vi "AP2_scope_viewer.vi"() -> ()   [LabVIEW 2023]
uses:
  <instrlib>/niScope/Controls/niScope vertical coupling.ctl
  <instrlib>/niScope/Controls/niScope trigger slope.ctl
  <instrlib>/niScope/Controls/niScope trigger source.ctl
panel:
  in  "Tab Control 2":enum32{"General", "Monitoring", "Advanced"}(tab)
  in  "stop":bool
  in  "Save C1 Trace":bool
  in  "Save C2 Trace":bool
  in  "C1 enabled":bool=TRUE caption="Enabled?"
  in  "C2 enabled":bool=TRUE caption="Enabled?"
  in  "Reset Summed Averages":bool
  in  "RT Avg Trace #":i32=10 min=1
  in  "Summed Trace #":i32=1000 min=1
  in  "Trigger delay / us":dbl caption="trigger delay" format="%.5f"
  in  "Probe Duration / us":dbl=100.0
  in  "Samples":i64(ring)=500000 items=["500 S"=500, "1 kS"=1000, "5 kS"=5000, "10 kS"=10000, "100 kS"=100000, "500 kS"=500000, "1 MS"=1000000, "2.5 MS"=2500000, "5MS"=5000000, "10 MS"=10000000, "20 MS"=20000000]
  in  "C1 Offset / V":dbl caption="vertical offset" format="%.4f"
  in  "C1 Coupling / V":T1=1 caption="vertical coupling" items=["AC", "DC", "Ground"]
  in  "C1 Range / V":dbl=0.1 caption="vertical range" min=0.1 max=5.0 step=0.1 format="%.2f"
  in  "C1 Attenuation":dbl=2.0 caption="probe attenuation" format="%.1f"
  in  "C1 Impedance":u32(ring)=2 caption="input impedance" items=["1 mega ohm"=0, "50 ohms"=2]
  in  "C2 Offset / V":dbl caption="vertical offset" format="%.4f"
  in  "C2 Range / V":dbl=1.0 caption="vertical range" min=0.1 max=5.0 step=0.1 format="%.2f"
  in  "C2 Attenuation":dbl=1.0 caption="probe attenuation" format="%.1f"
  in  "C2 Coupling / V":T1=1 caption="vertical coupling" items=["AC", "DC", "Ground"]
  in  "C2 Impedance":u32(ring)=2 caption="input impedance" items=["1 mega ohm"=0, "50 ohms"=2]
  in  "Trigger slope":T2 items=["Positive", "Negative"]
  in  "Trigger Source":string(combo)="VAL_PFI_0"
  in  "Load Scope Config":bool
  in  "Save Scope Config":bool
  out "Aqusition Time / ms":u32=100
  out "Aquisition Frequency / Hz":dbl=10.0
  out "Summed Avg  Exectuion Time / ms":u32=14
  out "Raw Data Processing  Exectuion Time / ms":u32=103
  out "RT Average Exectuion Time / ms":u32=18
  in  "Scope Channel":refnum<k15>="PXI1Slot2" caption="resource name"
  in  "Default Data Directory":path=path "" caption="start path"
  in  "C1 maximum input frequency / Hz":dbl=100.0 caption="max input frequency" format="%.2f"
  in  "Enforce realtime":bool=TRUE caption="enforce realtime"
  in  "C2 maximum input frequency / Hz":dbl caption="max input frequency" format="%.2f"
  in  "Load old conditions?":bool
  in  "Intercept":dbl
  in  "Gradient":dbl
  in  "Mass Conversion":bool
  in  "Tab Control 6":enum32{"Time Traces", "Mass Traces"}(tab)
  in  "Tab Control":T3(tab)=enum."Real Time Average Traces"
  in  "Tab Control 3":enum32{"Channel 1", "Channel 2"}(tab)
  out "Channel 2 Raw":waveform(dbl)(graph)
  out "Channel 1 Raw":waveform(dbl)(graph)
  in  "Tab Control 4":enum32{"Channel 1", "Channel 2"}(tab)
  out "Channel 1 RT Avg":waveform(dbl)(graph)
  out "Channel 2 RT Avg":waveform(dbl)(graph)
  in  "Tab Control 5":enum32{"Channel 1", "Channel 2"}(tab)
  out "Channel 1 Summed Avg":waveform(dbl)(graph)={"t0"=timestamp(3803903996.848833 s since 1904-01-01), "dt"=4e-10, "Y"=array[250000 elements]}
  out "Trace # (C1)":i32=1000
  out "Channel 2  Summed Avg":waveform(dbl)(graph)={"t0"=timestamp(3803903996.848833 s since 1904-01-01), "dt"=4e-10, "Y"=array[250000 elements]}
  out "Trace # (C2)":i32=1000
  in  "Tab Control 10":T3(tab)
  in  "Tab Control 7":enum32{"Channel 1", "Channel 2"}(tab)
  out "C1 Raw (mass)":cluster{dbl[], "Y":dbl[]}(graph)
  out "C2 Raw (mass)":cluster{dbl[], "Y":dbl[]}(graph)
  in  "Tab Control 8":enum32{"Channel 1", "Channel 2"}(tab)
  out "C1 RT avg (mass)":cluster{dbl[], "Y":dbl[]}(graph)
  out "C2 RT avg (mass)":cluster{dbl[], "Y":dbl[]}(graph)
  in  "Tab Control 9":enum32{"Channel 1", "Channel 2"}(tab)
  out "C1 Summed avg (mass)":cluster{dbl[], "Y":dbl[]}(graph)
  out "C2 Summed avg (mass)":cluster{dbl[], "Y":dbl[]}(graph)
  # "Triggering Controls"
  # "Vertical Controls"
  # "Horizontal Controls"
  # "Averaging Controls"
  # "Mass Conversion Controls"
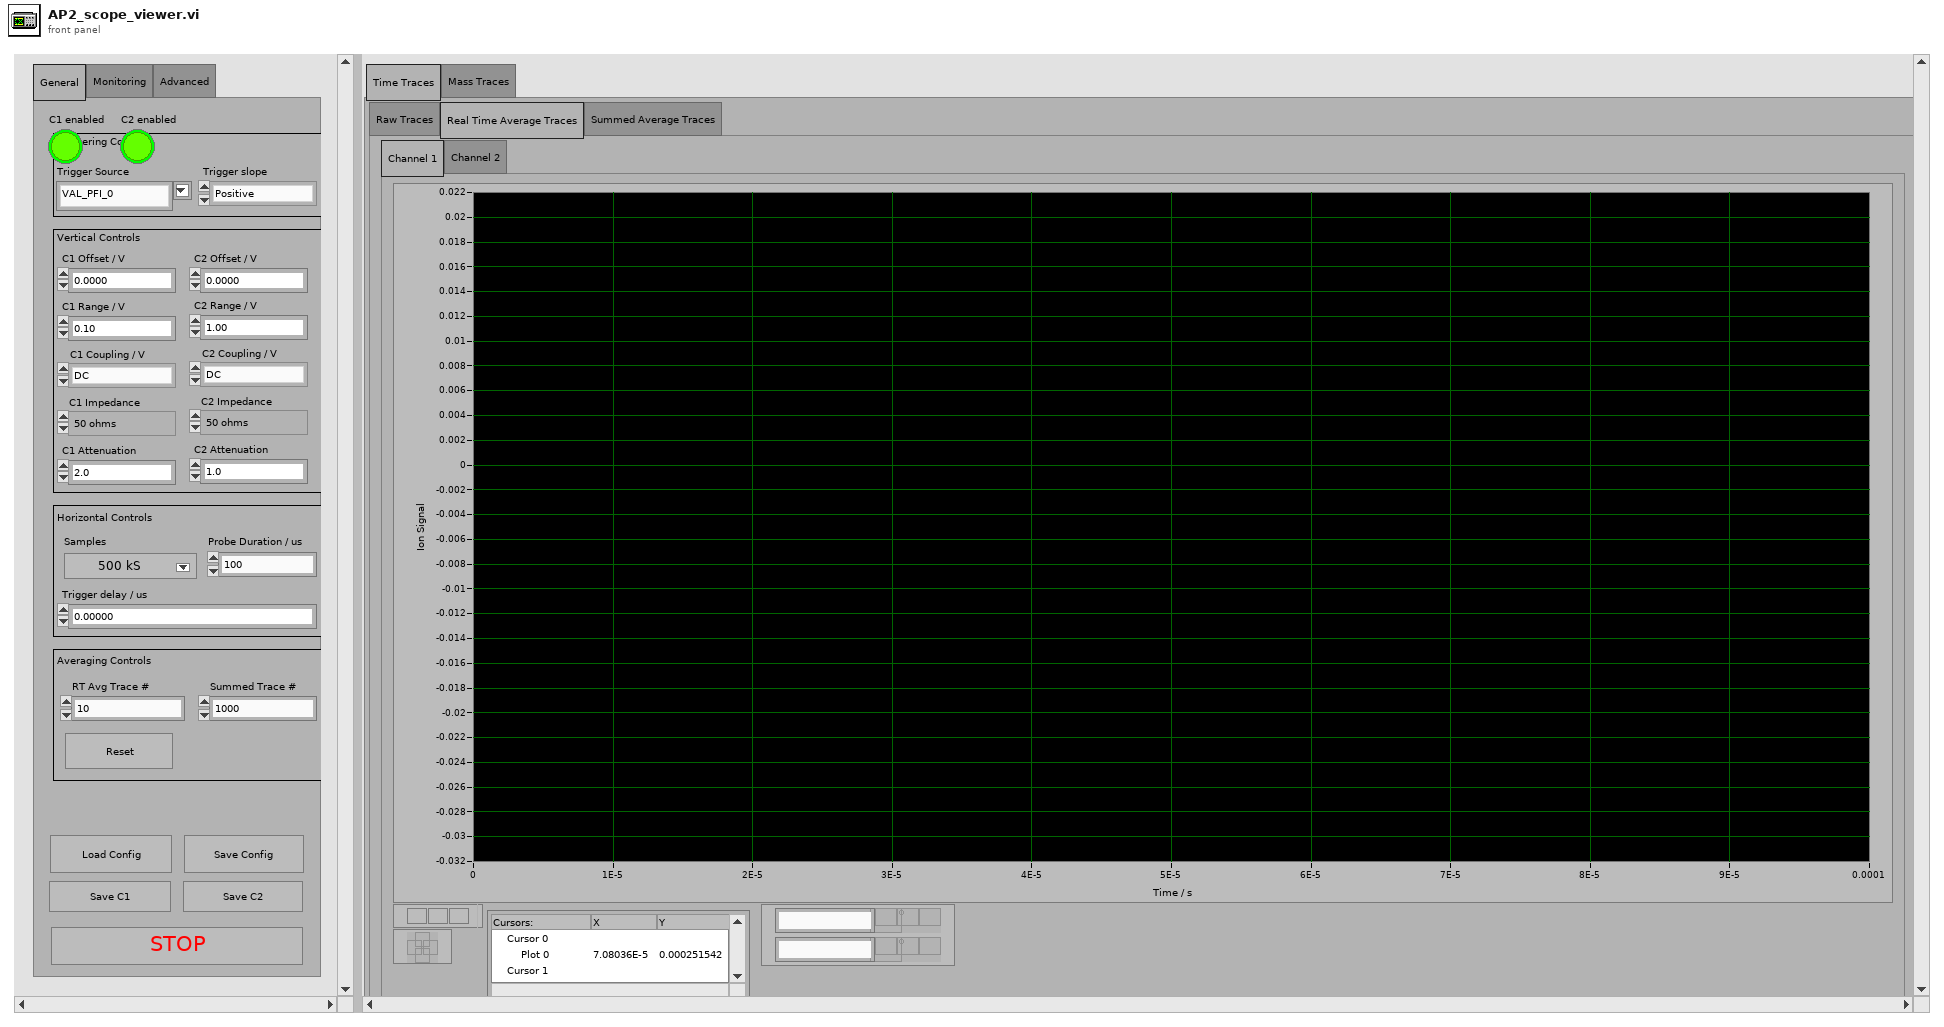
[diagram p1: front panel]
types:
  T1 = typedef "niScope vertical coupling.ctl" = i32
  T2 = typedef "niScope trigger slope.ctl" = i32
  T3 = enum32{"Raw Traces", "Real Time Average Traces", "Summed Average Traces"}
  T4 = cluster{"Trigger Source":refnum<vi>, "Trigger delay / us":refnum<vi>, "Trigger slope":refnum<vi>, "Probe Duration / us":refnum<vi>, "Samples":refnum<vi>, "Enforce realtime":refnum<vi>, "C2 Impedance":refnum<vi>, "C2 maximum input frequency / Hz":refnum<vi>, "C2 enabled":refnum<vi>, "C2 Coupling / V":refnum<vi>, "C2 Attenuation":refnum<vi>, "C2 Range / V":refnum<vi>, "C2 Offset / V":refnum<vi>, "C1 Impedance":refnum<vi>, "C1 maximum input frequency / Hz":refnum<vi>, "C1 enabled":refnum<vi>, "C1 Coupling / V":refnum<vi>, "C1 Attenuation":refnum<vi>, "C1 Range / V":refnum<vi>, "C1 Offset / V":refnum<vi>, "Scope Channel":refnum<vi>}
  T5 = cluster{"C1 Summed Waveform 2":waveform(dbl), "C1 Summed Waveform 2":waveform(dbl)}
  T6 = cluster{"Gradient":dbl, "Intercept":dbl, "RT Avg Trace #":i32, "Summed Avg Trace #":i32, "Mass Conversion":bool}
  T7 = typedef "niScope trigger source.ctl" = string
  T8 = cluster{"Scope Channel":refnum<k15>, "C1 vertical offset / V":dbl, "C1 vertical range / V":dbl, "C1 probe attenuation":dbl, "C1 vertical coupling / V":T1, "C1 enabled":bool, "C1 maximum input frequency / Hz":dbl, "C1 input impedance / ohms":u32, "C2 vertical offset / V":dbl, "C2 vertical range / V":dbl, "C2 probe attenuation":dbl, "C2 vertical coupling / V":T1, "C2 enabled":bool, "C2 maximum input frequency / Hz":dbl, "C2 input impedance / ohms":u32, "Enforce realtime":bool, "Samples":i64, "tmax / us ":dbl, "Trigger source":T7, "Trigger slope":T2, "Trigger delay / us":dbl}
  T9 = cluster{"queue out":refnum<queue>, "error out":errorcluster, "queue out":refnum<queue>, "error out":errorcluster, "queue out":refnum<queue>, "error out":errorcluster, "queue out":refnum<queue>, "error out":errorcluster}
  T10 = cluster{"queue out":refnum<queue>, "error out":errorcluster, "queue out":refnum<queue>, "error out":errorcluster}
  T11 = cluster{"output cluster":cluster{"wfm info":cluster{"actualSamples":i32, "absoluteInitialX":dbl, "relativeInitialX":dbl, "xIncrement":dbl, "offset":dbl, "gain":dbl, "reserved1":dbl, "reserved2":dbl}, "Offset WFm":waveform(dbl), bool}, "output cluster":cluster{"wfm info":cluster{"actualSamples":i32, "absoluteInitialX":dbl, "relativeInitialX":dbl, "xIncrement":dbl, "offset":dbl, "gain":dbl, "reserved1":dbl, "reserved2":dbl}, "Offset WFm":waveform(dbl), bool}}
  T12 = cluster{"Cycle Count In":i32, "Cycle Count In":i32}
  T13 = cluster{"output cluster":cluster{"wfm info":cluster{"actualSamples":i32, "absoluteInitialX":dbl, "relativeInitialX":dbl, "xIncrement":dbl, "offset":dbl, "gain":dbl, "reserved1":dbl, "reserved2":dbl}, "C1 Summed Waveform 2":waveform(dbl), bool}, "output cluster":cluster{"wfm info":cluster{"actualSamples":i32, "absoluteInitialX":dbl, "relativeInitialX":dbl, "xIncrement":dbl, "offset":dbl, "gain":dbl, "reserved1":dbl, "reserved2":dbl}, "C1 Summed Waveform 2":waveform(dbl), bool}, "C1 Mass Data":cluster{dbl, cluster{dbl, dbl}, cluster{dbl[], "Y":dbl[]}}, "C2 Mass Data":cluster{dbl, cluster{dbl, dbl}, cluster{dbl[], "Y":dbl[]}}}
  T14 = cluster{"offset":dbl, "C1 Summed Waveform 2":waveform(dbl)}
  T15 = cluster{"elements":cluster{"wfm info":cluster{"actualSamples":i32, "absoluteInitialX":dbl, "relativeInitialX":dbl, "xIncrement":dbl, "offset":dbl, "gain":dbl, "reserved1":dbl, "reserved2":dbl}, "Offset WFm":waveform(dbl), bool}[], "elements":cluster{"wfm info":cluster{"actualSamples":i32, "absoluteInitialX":dbl, "relativeInitialX":dbl, "xIncrement":dbl, "offset":dbl, "gain":dbl, "reserved1":dbl, "reserved2":dbl}, "Offset WFm":waveform(dbl), bool}[]}
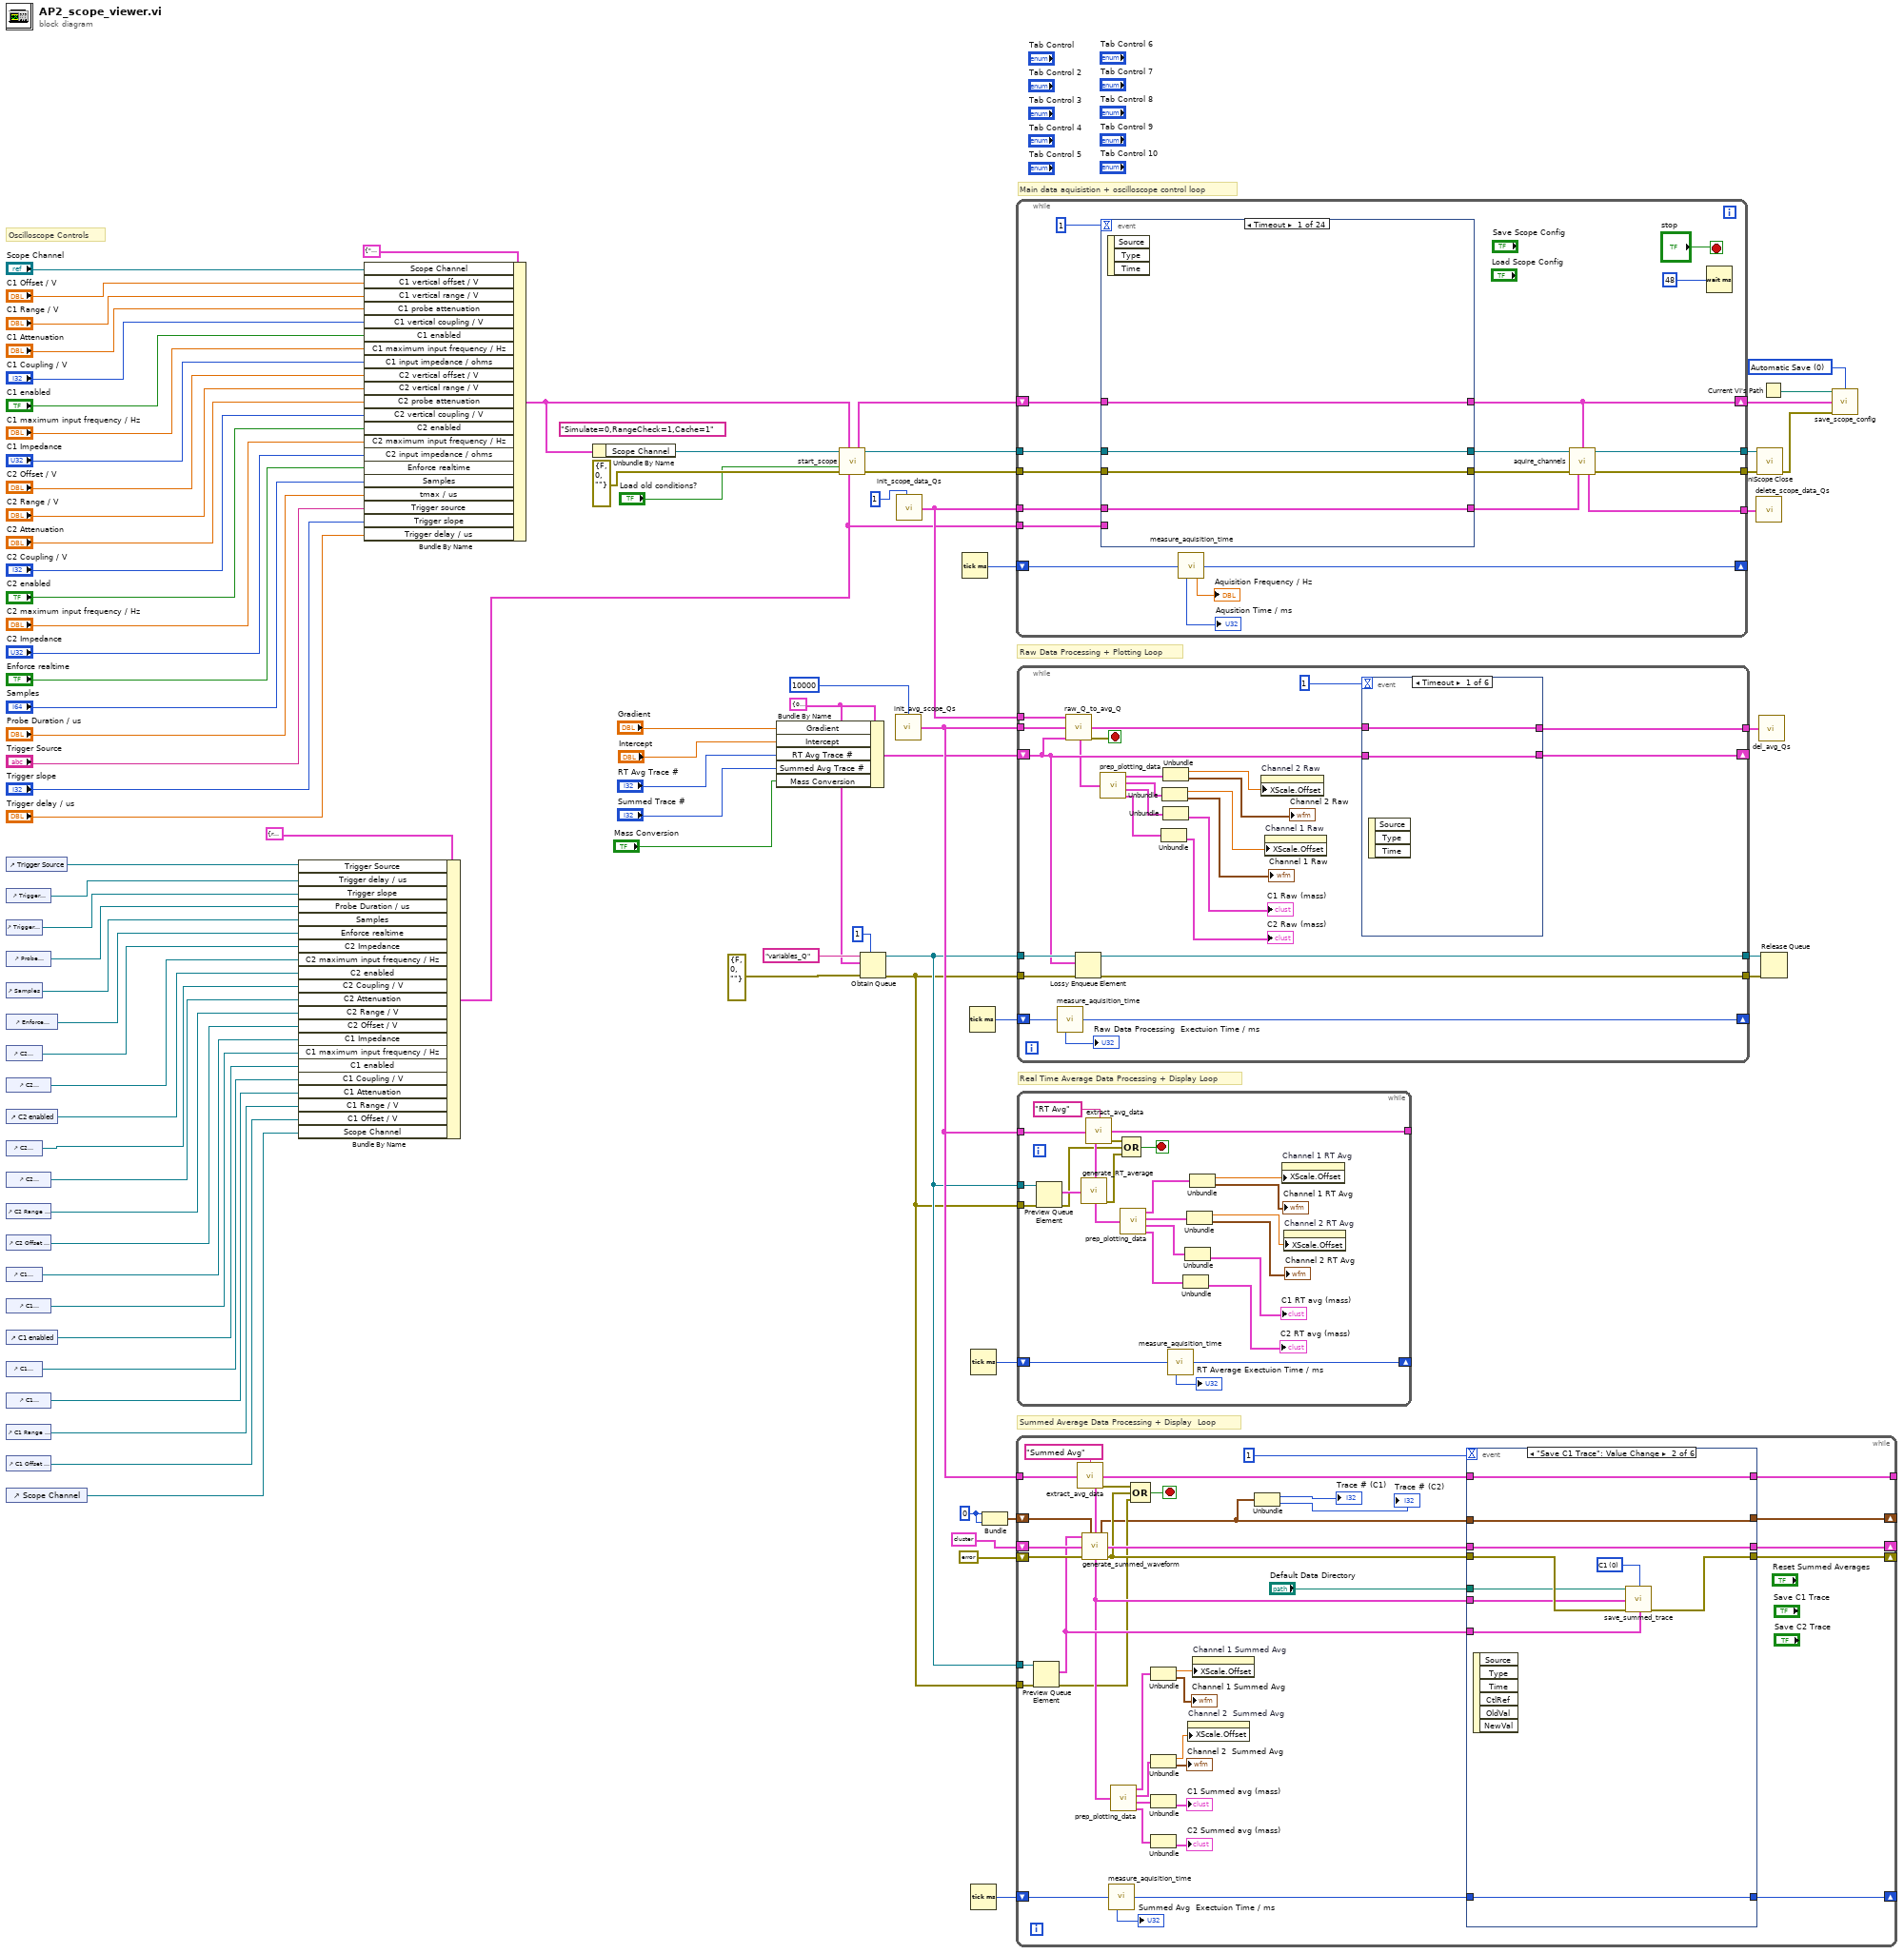
[diagram p0: block diagram]
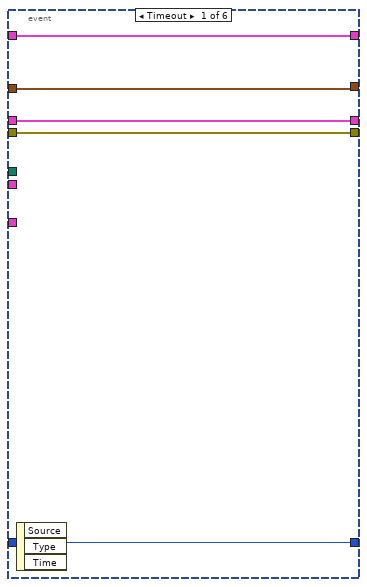
[diagram p2: hidden frame]
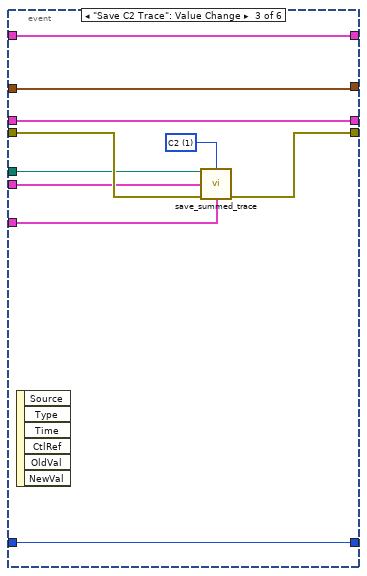
[diagram p3: hidden frame]
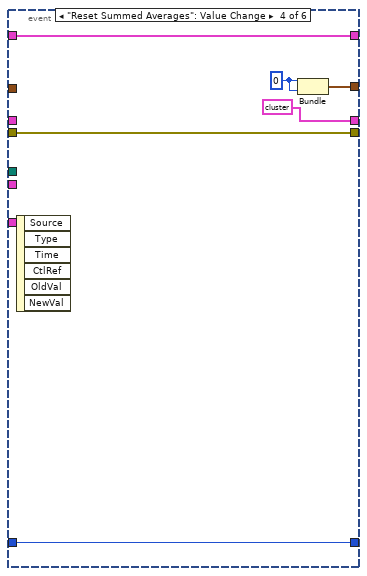
[diagram p4: hidden frame]
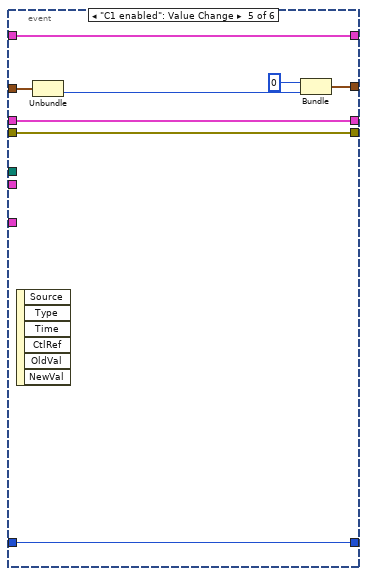
[diagram p5: hidden frame]
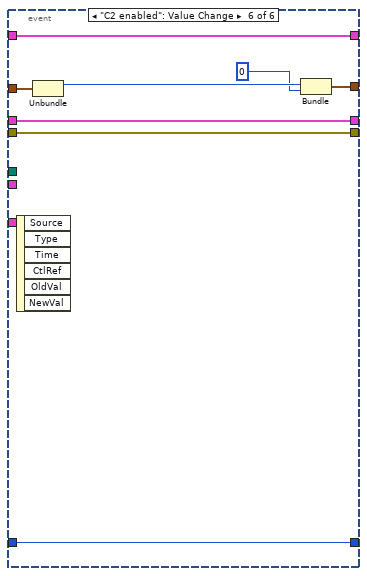
[diagram p6: hidden frame]
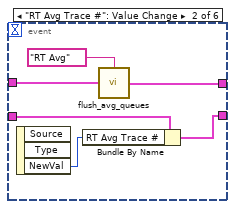
[diagram p7: hidden frame]
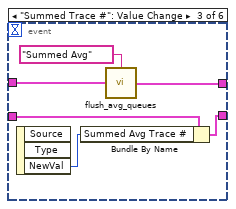
[diagram p8: hidden frame]
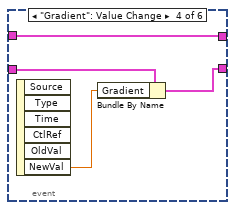
[diagram p9: hidden frame]
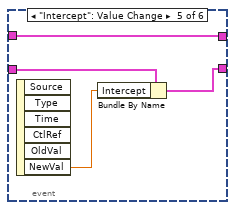
[diagram p10: hidden frame]
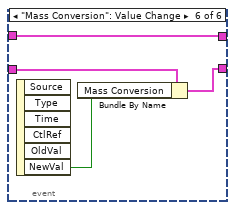
[diagram p11: hidden frame]
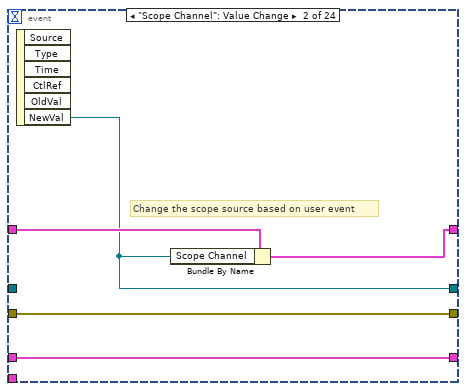
[diagram p12: hidden frame]
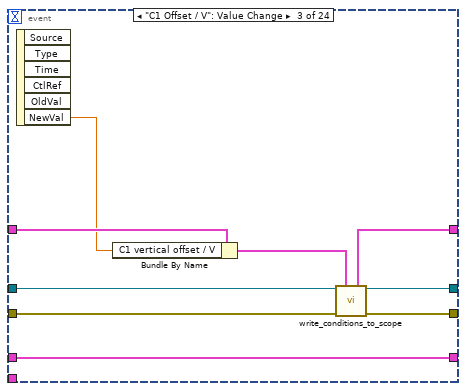
[diagram p13: hidden frame]
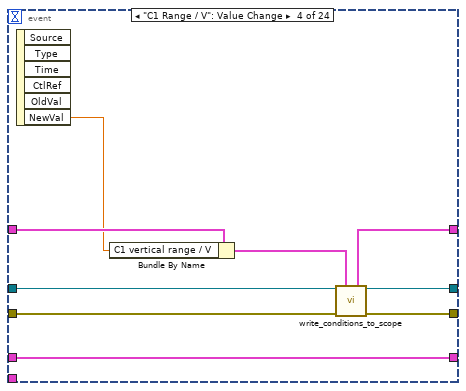
[diagram p14: hidden frame]
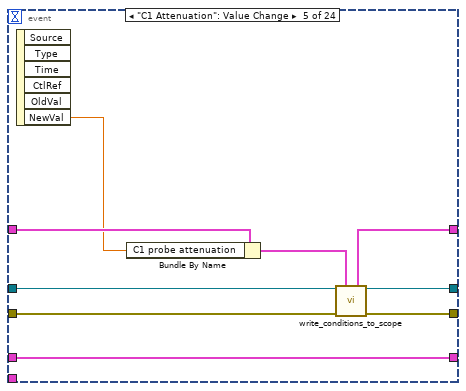
[diagram p15: hidden frame]
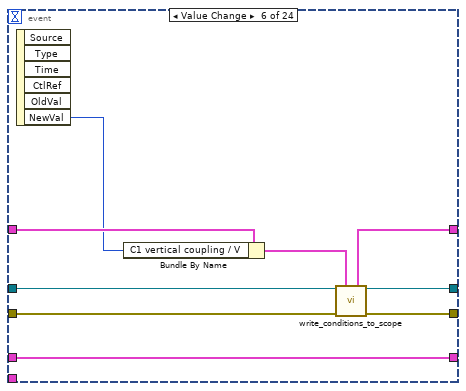
[diagram p16: hidden frame]
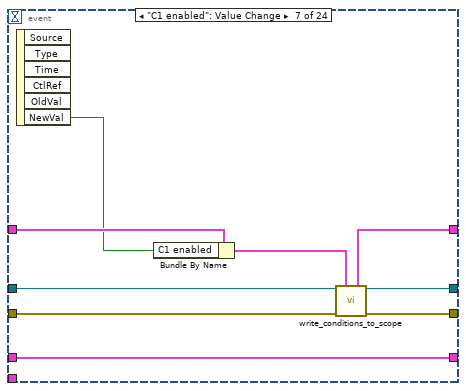
[diagram p17: hidden frame]
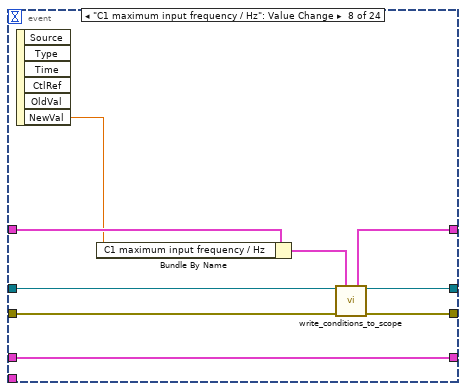
[diagram p18: hidden frame]
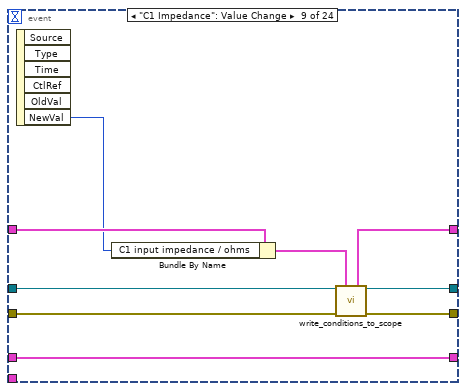
[diagram p19: hidden frame]
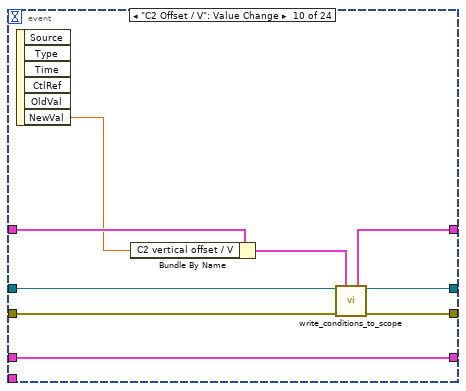
[diagram p20: hidden frame]
diagram:
  w31 = u16 0 items=["Automatic Save", "Custom File"] ("Save File Type")
  w41 = 0
  w49 = T6 {"Gradient"=0.0, "Intercept"=0.0, "RT Avg Trace #"=0, "Summed Avg Trace #"=0, "Mass Conversion"=FALSE}
  (unwired) "Simulate=0,RangeCheck=1,Cache=1" ("option string")
  # "Summed Average Data Processing + Display  Loop"
  # "Real Time Average Data Processing + Display Loop"
  # "Oscilloscope Controls"
  # "Raw Data Processing + Plotting Loop"
  # "Main data aquisistion + oscilloscope control loop"
  n1 = control-ref of="Trigger Source"() -> (w23:refnum<vi>)
  n2 = control-ref of="Trigger delay / us"() -> (w21:refnum<vi>)
  n3 = control-ref of="Trigger slope"() -> (w20:refnum<vi>)
  n4 = control-ref of="Probe Duration / us"() -> (w19:refnum<vi>)
  n5 = control-ref of="Samples"() -> (w18:refnum<vi>)
  n6 = control-ref of="Enforce realtime"() -> (w17:refnum<vi>)
  n7 = control-ref of="C2 Impedance"() -> (w16:refnum<vi>)
  n8 = control-ref of="C2 maximum input frequency / Hz"() -> (w15:refnum<vi>)
  n9 = control-ref of="C2 enabled"() -> (w14:refnum<vi>)
  n10 = control-ref of="C2 Coupling / V"() -> (w13:refnum<vi>)
  n11 = control-ref of="C2 Attenuation"() -> (w12:refnum<vi>)
  n12 = control-ref of="C2 Range / V"() -> (w11:refnum<vi>)
  n13 = control-ref of="C2 Offset / V"() -> (w10:refnum<vi>)
  n14 = control-ref of="C1 Impedance"() -> (w9:refnum<vi>)
  n15 = control-ref of="C1 maximum input frequency / Hz"() -> (w8:refnum<vi>)
  n16 = control-ref of="C1 enabled"() -> (w7:refnum<vi>)
  n17 = control-ref of="C1 Coupling / V"() -> (w6:refnum<vi>)
  n18 = control-ref of="C1 Attenuation"() -> (w5:refnum<vi>)
  n19 = control-ref of="C1 Range / V"() -> (w4:refnum<vi>)
  n20 = control-ref of="C1 Offset / V"() -> (w3:refnum<vi>)
  n21 = control-ref of="Scope Channel"() -> (w2:refnum<vi>)
  n22 = Bundle By Name(cluster=T4 {"Trigger Source"=refnum, "Trigger delay / us"=refnum, "Trigger slope"=refnum, "Probe Duration / us"=refnum, "Samples"=refnum, "Enforce realtime"=refnum, "C2 Impedance"=refnum, "C2 maximum input frequency / Hz"=refnum, "C2 enabled"=refnum, "C2 Coupling / V"=refnum, "C2 Attenuation"=refnum, "C2 Range / V"=refnum, "C2 Offset / V"=refnum, "C1 Impedance"=refnum, "C1 maximum input frequency / Hz"=refnum, "C1 enabled"=refnum, "C1 Coupling / V"=refnum, "C1 Attenuation"=refnum, "C1 Range / V"=refnum, "C1 Offset / V"=refnum, "Scope Channel"=refnum}, "Trigger Source"=w23, "Trigger delay / us"=w21, "Trigger slope"=w20, "Probe Duration / us"=w19, "Samples"=w18, "Enforce realtime"=w17, "C2 Impedance"=w16, "C2 maximum input frequency / Hz"=w15, "C2 enabled"=w14, "C2 Coupling / V"=w13, "C2 Attenuation"=w12, "C2 Range / V"=w11, "C2 Offset / V"=w10, "C1 Impedance"=w9, "C1 maximum input frequency / Hz"=w8, "C1 enabled"=w7, "C1 Coupling / V"=w6, "C1 Attenuation"=w5, "C1 Range / V"=w4, "C1 Offset / V"=w3, "Scope Channel"=w2) -> (w1:T4)
  n23 = Bundle By Name(cluster=T8 {"Scope Channel"="", "C1 vertical offset / V"=0.0, "C1 vertical range / V"=5.0, "C1 probe attenuation"=1.0, "C1 vertical coupling / V"=1, "C1 enabled"=TRUE, "C1 maximum input frequency / Hz"=0.0, "C1 input impedance / ohms"=0, "C2 vertical offset / V"=0.0, "C2 vertical range / V"=5.0, "C2 probe attenuation"=1.0, "C2 vertical coupling / V"=1, "C2 enabled"=TRUE, "C2 maximum input frequency / Hz"=0.0, "C2 input impedance / ohms"=0, "Enforce realtime"=TRUE, "Samples"=0, "tmax / us "=0.0, "Trigger source"="0", "Trigger slope"=0, "Trigger delay / us"=0.0}, "Scope Channel"="Scope Channel", "C1 vertical offset / V"="C1 Offset / V", "C1 vertical range / V"="C1 Range / V", "C1 probe attenuation"="C1 Attenuation", "C1 vertical coupling / V"="C1 Coupling / V", "C1 enabled"="C1 enabled", "C1 maximum input frequency / Hz"="C1 maximum input frequency / Hz", "C1 input impedance / ohms"="C1 Impedance", "C2 vertical offset / V"="C2 Offset / V", "C2 vertical range / V"="C2 Range / V", "C2 probe attenuation"="C2 Attenuation", "C2 vertical coupling / V"="C2 Coupling / V", "C2 enabled"="C2 enabled", "C2 maximum input frequency / Hz"="C2 maximum input frequency / Hz", "C2 input impedance / ohms"="C2 Impedance", "Enforce realtime"="Enforce realtime", "Samples"="Samples", "tmax / us"="Probe Duration / us", "Trigger source"="Trigger Source", "Trigger slope"="Trigger slope", "Trigger delay / us"="Trigger delay / us") -> (w27:T8)
  n24 = Unbundle By Name(w27) -> ("Scope Channel"=w30:refnum<k15>)
  n25 = Bundle By Name(cluster=w49, "Gradient"="Gradient", "Intercept"="Intercept", "RT Avg Trace #"="RT Avg Trace #", "Summed Avg Trace #"="Summed Trace #", "Mass Conversion"="Mass Conversion") -> (w53:T6)
  n26 = call "start_scope.vi"("resource name"=w30, "Controls cluster"=w27, "Load old conditions"="Load old conditions?", "error in"=errorcluster {"status"=FALSE, "code"=0, "source"=""}, "Controls References Cluster In"=w1) -> ("Controls cluster out"=w26:T8, "instrument handle out"=w29:refnum<k15>, "error out"=w28:errorcluster)  [unwired: 7 in, 1 out]
  n27 = Obtain Queue(max queue size (-1, unlimited)=1, name (unnamed)="variables_Q", element data type=w49, error in (no error)=errorcluster {"status"=FALSE, "code"=0, "source"=""}) -> (queue out=w39:refnum<queue>, error out=w38:errorcluster)  [unwired: 1 in, 1 out]
  n28 = call "init_avg_scope_Qs.vi"("max summed queue size (-1, unlimited)"=10000 ("max queue size (-1, unlimited)")) -> ("avg_Q_data"=w57:T9)  [unwired: 14 in]
  n29 = call "init_scope_data_Qs.vi"("max queue size (-1, unlimited)"=1) -> ("scope Q data"=w64:T10)  [unwired: 5 in]
  n30 = Tick Count (ms)() -> (millisecond timer value=w86:u32)
  n31 = Tick Count (ms)() -> (millisecond timer value=w35:u32)
  n32 = Tick Count (ms)() -> (millisecond timer value=w45:u32)
  n33 = Tick Count (ms)() -> (millisecond timer value=w37:u32)
  n34 = Bundle(w41, w41) -> (w40:cluster{i32, i32})  [unwired: 1 in]
  n35 = while {
    shift-right: [w102] -> _
    shift-left: w86 -> [w103]
    tunnel: w29 -> [w96]
    tunnel: w28 -> [w94]
    tunnel: [w101] -> w66
    tunnel: [w100] -> w65
    tunnel: w64 -> [w93]
    tunnel: [w97] -> w61
    shift-right: [w88] -> w33
    shift-left: w26 -> [w89]
    tunnel: w1 -> [w87]
    stop <- "stop" stop-if-true
    n36 = event shown="[0] Timeout" {
      selector: _ -> [_ _ _ _ _ _ _ _ _ _ _ _ _ _ _ _ _ _ _ _ _ _ _ _]
      dyn-events: _ -> [_ _ _ _ _ _ _ _ _ _ _ _ _ _ _ _ _ _ _ _ _ _ _ _]
      timeout: 1 -> [_ _ _ _ _ _ _ _ _ _ _ _ _ _ _ _ _ _ _ _ _ _ _ _]
      tunnel: w96 -> [w109 _ w121 w130 w139 w148 w157 w166 w175 w184 w193 w202 w211 w220 w229 w238 w247 w256 w265 w274 w283 w292 w302 w309]
      tunnel: w94 -> [w108 w114 w120 w129 w138 w147 w156 w165 w174 w183 w192 w201 w210 w219 w228 w237 w246 w255 w264 w273 w282 w291 w298 w305]
      tunnel: w93 -> [w107 w113 w115 w124 w133 w142 w151 w160 w169 w178 w187 w196 w205 w214 w223 w232 w241 w250 w259 w269 w277 w286 w301 w310]
      tunnel: [w109 w110 w123 w132 w141 w150 w159 w168 w177 w186 w195 w204 w213 w222 w231 w240 w249 w258 w267 w276 w285 w294 w302 w309] -> w92
      tunnel: [w108 w114 w122 w131 w140 w149 w158 w167 w176 w185 w194 w203 w212 w221 w230 w239 w248 w257 w266 w275 w284 w293 w297 w304] -> w91
      tunnel: [w107 w113 w115 w124 w133 w142 w151 w160 w169 w178 w187 w196 w205 w214 w223 w232 w241 w250 w259 w269 w277 w286 w301 w310] -> w90
      tunnel: w89 -> [w106 w112 w118 w127 w136 w145 w154 w163 w172 w181 w190 w199 w208 w217 w226 w235 w244 w253 w262 w271 w280 w289 w300 w306]
      tunnel: [w106 w111 w119 w128 w137 w146 w155 w164 w173 w182 w191 w200 w209 w218 w227 w236 w245 w254 w263 w272 w281 w290 w299 w306] -> w88
      tunnel: w87 -> [_ _ _ _ _ _ _ _ _ _ _ _ _ _ _ _ _ _ _ _ _ _ _ w303]
      event Timeout {
        n37 = event-data() -> ()  [unwired: 1 in, 3 out]
      }
      event "Scope Channel": Value Change {
        # "Change the scope source based on user event"
        n38 = event-data() -> ("NewVal"=w110:refnum<k15>)  [unwired: 1 in, 5 out]
        n39 = Bundle By Name(cluster=w112, "Scope Channel"=w110) -> (w111:T8)
      }
      event "C1 Offset / V": Value Change {
        n40 = event-data() -> ("NewVal"=w116:dbl)  [unwired: 1 in, 5 out]
        n41 = Bundle By Name(cluster=w118, "C1 vertical offset / V"=w116) -> (w117:T8)
        n42 = call "write_conditions_to_scope.vi"("instrument handle"=w121, "Controls Cluster In"=w117, "error in"=w120) -> ("Controls Cluster Out"=w119:T8, "instrument handle out"=w123:refnum<k15>, "error out"=w122:errorcluster)  [unwired: 10 in]
      }
      event "C1 Range / V": Value Change {
        n43 = event-data() -> ("NewVal"=w125:dbl)  [unwired: 1 in, 5 out]
        n44 = Bundle By Name(cluster=w127, "C1 vertical range / V"=w125) -> (w126:T8)
        n45 = call "write_conditions_to_scope.vi"("instrument handle"=w130, "Controls Cluster In"=w126, "error in"=w129) -> ("Controls Cluster Out"=w128:T8, "instrument handle out"=w132:refnum<k15>, "error out"=w131:errorcluster)  [unwired: 10 in]
      }
      event "C1 Attenuation": Value Change {
        n46 = event-data() -> ("NewVal"=w134:dbl)  [unwired: 1 in, 5 out]
        n47 = Bundle By Name(cluster=w136, "C1 probe attenuation"=w134) -> (w135:T8)
        n48 = call "write_conditions_to_scope.vi"("instrument handle"=w139, "Controls Cluster In"=w135, "error in"=w138) -> ("Controls Cluster Out"=w137:T8, "instrument handle out"=w141:refnum<k15>, "error out"=w140:errorcluster)  [unwired: 10 in]
      }
      event Value Change {
        n49 = event-data() -> ("NewVal"=w143:T1)  [unwired: 1 in, 5 out]
        n50 = Bundle By Name(cluster=w145, "C1 vertical coupling / V"=w143) -> (w144:T8)
        n51 = call "write_conditions_to_scope.vi"("instrument handle"=w148, "Controls Cluster In"=w144, "error in"=w147) -> ("Controls Cluster Out"=w146:T8, "instrument handle out"=w150:refnum<k15>, "error out"=w149:errorcluster)  [unwired: 10 in]
      }
      event "C1 enabled": Value Change {
        n52 = event-data() -> ("NewVal"=w152:bool)  [unwired: 1 in, 5 out]
        n53 = Bundle By Name(cluster=w154, "C1 enabled"=w152) -> (w153:T8)
        n54 = call "write_conditions_to_scope.vi"("instrument handle"=w157, "Controls Cluster In"=w153, "error in"=w156) -> ("Controls Cluster Out"=w155:T8, "instrument handle out"=w159:refnum<k15>, "error out"=w158:errorcluster)  [unwired: 10 in]
      }
      event "C1 maximum input frequency / Hz": Value Change {
        n55 = event-data() -> ("NewVal"=w161:dbl)  [unwired: 1 in, 5 out]
        n56 = Bundle By Name(cluster=w163, "C1 maximum input frequency / Hz"=w161) -> (w162:T8)
        n57 = call "write_conditions_to_scope.vi"("instrument handle"=w166, "Controls Cluster In"=w162, "error in"=w165) -> ("Controls Cluster Out"=w164:T8, "instrument handle out"=w168:refnum<k15>, "error out"=w167:errorcluster)  [unwired: 10 in]
      }
      event "C1 Impedance": Value Change {
        n58 = event-data() -> ("NewVal"=w170:u32)  [unwired: 1 in, 5 out]
        n59 = Bundle By Name(cluster=w172, "C1 input impedance / ohms"=w170) -> (w171:T8)
        n60 = call "write_conditions_to_scope.vi"("instrument handle"=w175, "Controls Cluster In"=w171, "error in"=w174) -> ("Controls Cluster Out"=w173:T8, "instrument handle out"=w177:refnum<k15>, "error out"=w176:errorcluster)  [unwired: 10 in]
      }
      event "C2 Offset / V": Value Change {
        n61 = event-data() -> ("NewVal"=w179:dbl)  [unwired: 1 in, 5 out]
        n62 = Bundle By Name(cluster=w181, "C2 vertical offset / V"=w179) -> (w180:T8)
        n63 = call "write_conditions_to_scope.vi"("instrument handle"=w184, "Controls Cluster In"=w180, "error in"=w183) -> ("Controls Cluster Out"=w182:T8, "instrument handle out"=w186:refnum<k15>, "error out"=w185:errorcluster)  [unwired: 10 in]
      }
      event "C2 Range / V": Value Change {
        n64 = event-data() -> ("NewVal"=w188:dbl)  [unwired: 1 in, 5 out]
        n65 = Bundle By Name(cluster=w190, "C2 vertical range / V"=w188) -> (w189:T8)
        n66 = call "write_conditions_to_scope.vi"("instrument handle"=w193, "Controls Cluster In"=w189, "error in"=w192) -> ("Controls Cluster Out"=w191:T8, "instrument handle out"=w195:refnum<k15>, "error out"=w194:errorcluster)  [unwired: 10 in]
      }
      event "C2 Attenuation": Value Change {
        n67 = event-data() -> ("NewVal"=w197:dbl)  [unwired: 1 in, 5 out]
        n68 = Bundle By Name(cluster=w199, "C2 probe attenuation"=w197) -> (w198:T8)
        n69 = call "write_conditions_to_scope.vi"("instrument handle"=w202, "Controls Cluster In"=w198, "error in"=w201) -> ("Controls Cluster Out"=w200:T8, "instrument handle out"=w204:refnum<k15>, "error out"=w203:errorcluster)  [unwired: 10 in]
      }
      event Value Change {
        n70 = event-data() -> ("NewVal"=w206:T1)  [unwired: 1 in, 5 out]
        n71 = Bundle By Name(cluster=w208, "C2 vertical coupling / V"=w206) -> (w207:T8)
        n72 = call "write_conditions_to_scope.vi"("instrument handle"=w211, "Controls Cluster In"=w207, "error in"=w210) -> ("Controls Cluster Out"=w209:T8, "instrument handle out"=w213:refnum<k15>, "error out"=w212:errorcluster)  [unwired: 10 in]
      }
      event "C2 enabled": Value Change {
        n73 = event-data() -> ("NewVal"=w215:bool)  [unwired: 1 in, 5 out]
        n74 = Bundle By Name(cluster=w217, "C2 enabled"=w215) -> (w216:T8)
        n75 = call "write_conditions_to_scope.vi"("instrument handle"=w220, "Controls Cluster In"=w216, "error in"=w219) -> ("Controls Cluster Out"=w218:T8, "instrument handle out"=w222:refnum<k15>, "error out"=w221:errorcluster)  [unwired: 10 in]
      }
      event "C2 maximum input frequency / Hz": Value Change {
        n76 = event-data() -> ("NewVal"=w224:dbl)  [unwired: 1 in, 5 out]
        n77 = Bundle By Name(cluster=w226, "C2 maximum input frequency / Hz"=w224) -> (w225:T8)
        n78 = call "write_conditions_to_scope.vi"("instrument handle"=w229, "Controls Cluster In"=w225, "error in"=w228) -> ("Controls Cluster Out"=w227:T8, "instrument handle out"=w231:refnum<k15>, "error out"=w230:errorcluster)  [unwired: 10 in]
      }
      event "C2 Impedance": Value Change {
        n79 = event-data() -> ("NewVal"=w233:u32)  [unwired: 1 in, 5 out]
        n80 = Bundle By Name(cluster=w235, "C2 input impedance / ohms"=w233) -> (w234:T8)
        n81 = call "write_conditions_to_scope.vi"("instrument handle"=w238, "Controls Cluster In"=w234, "error in"=w237) -> ("Controls Cluster Out"=w236:T8, "instrument handle out"=w240:refnum<k15>, "error out"=w239:errorcluster)  [unwired: 10 in]
      }
      event "Enforce realtime": Value Change {
        n82 = event-data() -> ("NewVal"=w242:bool)  [unwired: 1 in, 5 out]
        n83 = Bundle By Name(cluster=w244, "Enforce realtime"=w242) -> (w243:T8)
        n84 = call "write_conditions_to_scope.vi"("instrument handle"=w247, "Controls Cluster In"=w243, "error in"=w246) -> ("Controls Cluster Out"=w245:T8, "instrument handle out"=w249:refnum<k15>, "error out"=w248:errorcluster)  [unwired: 10 in]
      }
      event "Samples": Value Change {
        n85 = event-data() -> ("NewVal"=w251:i64)  [unwired: 1 in, 5 out]
        n86 = Bundle By Name(cluster=w253, "Samples"=w251) -> (w252:T8)
        n87 = call "write_conditions_to_scope.vi"("instrument handle"=w256, "Controls Cluster In"=w252, "error in"=w255) -> ("Controls Cluster Out"=w254:T8, "instrument handle out"=w258:refnum<k15>, "error out"=w257:errorcluster)  [unwired: 10 in]
      }
      event "Probe Duration / us": Value Change {
        n88 = event-data() -> ("NewVal"=w260:dbl)  [unwired: 1 in, 5 out]
        n89 = Bundle By Name(cluster=w262, "tmax / us"=w260) -> (w261:T8)
        n90 = call "write_conditions_to_scope.vi"("instrument handle"=w265, "Controls Cluster In"=w261, "error in"=w264) -> ("Controls Cluster Out"=w263:T8, "instrument handle out"=w267:refnum<k15>, "error out"=w266:errorcluster)  [unwired: 10 in]
      }
      event "Trigger Source": Value Change {
        n91 = event-data() -> ("NewVal"=w268:string)  [unwired: 1 in, 5 out]
        n92 = Bundle By Name(cluster=w271, "Trigger source"=w268) -> (w270:T8)
        n93 = call "write_conditions_to_scope.vi"("instrument handle"=w274, "Controls Cluster In"=w270, "error in"=w273) -> ("Controls Cluster Out"=w272:T8, "instrument handle out"=w276:refnum<k15>, "error out"=w275:errorcluster)  [unwired: 10 in]
      }
      event Value Change {
        n94 = event-data() -> ("NewVal"=w278:T2)  [unwired: 1 in, 5 out]
        n95 = Bundle By Name(cluster=w280, "Trigger slope"=w278) -> (w279:T8)
        n96 = call "write_conditions_to_scope.vi"("instrument handle"=w283, "Controls Cluster In"=w279, "error in"=w282) -> ("Controls Cluster Out"=w281:T8, "instrument handle out"=w285:refnum<k15>, "error out"=w284:errorcluster)  [unwired: 10 in]
      }
      event "Trigger delay / us": Value Change {
        n97 = event-data() -> ("NewVal"=w287:dbl)  [unwired: 1 in, 5 out]
        n98 = Bundle By Name(cluster=w289, "Trigger delay / us"=w287) -> (w288:T8)
        n99 = call "write_conditions_to_scope.vi"("instrument handle"=w292, "Controls Cluster In"=w288, "error in"=w291) -> ("Controls Cluster Out"=w290:T8, "instrument handle out"=w294:refnum<k15>, "error out"=w293:errorcluster)  [unwired: 10 in]
      }
      event "Save Scope Config": Value Change {
        w295 = u16 1 items=["Automatic Save", "Custom File"] ("Save File Type")
        n100 = event-data() -> ()  [unwired: 1 in, 6 out]
        n101 = Current VI's Path() -> (path=w296:path)
        n102 = call "save_scope_config.vi"("Current VI's Path"=w296, "Save File Type"=w295, "Controls cluster"=w300, "error in"=w298) -> ("Controls cluster out"=w299:T8, "error out"=w297:errorcluster)  [unwired: 10 in]
      }
      event "Load Scope Config": Value Change {
        w307 = u16 1 items=["Automatic Load", "Custom File"] ("Load File Type")
        n103 = event-data() -> ()  [unwired: 1 in, 6 out]
        n104 = Current VI's Path() -> (path=w308:path)
        n105 = call "load_scope_config.vi"("Load File Type"=w307, "error in"=w305, "Controls References Cluster In"=w303, "Controls cluster"=w306, "Current VI's Path"=w308) -> ("error out"=w304:errorcluster)  [unwired: 4 in, 2 out]
      }
    }
    n106 = call "measure_aquisition_time.vi"("Old Time / ms"=w103) -> ("New Time / ms"=w102:u32, "Aqusition Time / ms"=→"Aqusition Time / ms":u32, "Aquisition Frequency / Hz"=→"Aquisition Frequency / Hz":dbl)  [unwired: 12 in]
    n107 = call "aquire_channels.vi"("instrument handle"=w92, "Controls Cluster"=w88, "error in"=w91, "scope Q data in"=w90) -> ("instrument handle out"=w101:refnum<k15>, "scope Q data out"=w97:T10, "error out"=w100:errorcluster)  [unwired: 9 in]
    n108 = Wait (ms)(milliseconds to wait=u32 48) -> ()  [unwired: 1 out]
  }
  n109 = while {
    tunnel: w57 -> [w349]
    tunnel: [w346] -> _
    shift-right: [w320] -> _
    shift-left: errorcluster {"status"=FALSE, "code"=0, "source"=""} ("error out") -> [w343]
    shift-right: [w341] -> _
    shift-left: w40 -> [w342]
    tunnel: w39 -> [w334]
    tunnel: w38 -> [w333]
    shift-right: [w332] -> _
    shift-left: T5 {"C1 Summed Waveform 2"={"t0"=timestamp(0 s since 1904-01-01), "dt"=1.0, "Y"=[]}, "C1 Summed Waveform 2"={"t0"=timestamp(0 s since 1904-01-01), "dt"=1.0, "Y"=[]}} ("Summed WFms In") -> [w335]
    shift-right: [w336] -> _
    shift-left: w37 -> [w338]
    stop <- w317 stop-if-true
    n110 = Preview Queue Element(queue=w334, error in (no error)=w333) -> (element=w319:T6, error out=w314:errorcluster)  [unwired: 1 in, 2 out]
    n111 = call "extract_avg_data.vi"("Combo Box"="Summed Avg", "avg_Q_data in"=w349) -> ("avg_Q_data out"=w347:T9, "Summed Avg Data"=w344:T11, "error out"=w316:errorcluster)  [unwired: 10 in, 1 out]
    n112 = call "generate_summed_waveform.vi"("Variables Cluster"=w319, "Cycle Count Cluster In"=w342, "Summed Avg Data"=w344, "Summed WFms In"=w335, "error in (no error)"=w343) -> ("Cycle Count Cluster Out"=w313:T12, "Summed WFms Out"=w340:T5, "Complete Data Out"=w318:T13, "error out"=w315:errorcluster)  [unwired: 7 in]
    n113 = call "measure_aquisition_time.vi"("Old Time / ms"=w338) -> ("New Time / ms"=w337:u32, "Aqusition Time / ms"=→"Summed Avg  Exectuion Time / ms":u32)  [unwired: 12 in, 1 out]
    n114 = call "prep_plotting_data.vi"("Plotting Data"=w318) -> ("C1 (time)"=w330:T14, "C2 (time)"=w327:T14, "C1 (mass)"=w324:cluster{dbl, cluster{dbl[], "Y":dbl[]}}, "C2 (mass)"=w322:cluster{dbl, cluster{dbl[], "Y":dbl[]}})  [unwired: 4 in]
    n115 = Compound Arithmetic op=OR(w316, w315, w314) -> (w317:bool)
    n116 = Unbundle(w330) -> ("offset"=w329:dbl, "C1 Summed Waveform 2"=→"Channel 1 Summed Avg":waveform(dbl))
    n117 = Unbundle(w327) -> ("offset"=w326:dbl, "C1 Summed Waveform 2"=→"Channel 2  Summed Avg":waveform(dbl))
    n118 = Unbundle(w324) -> (→"C1 Summed avg (mass)":cluster{dbl[], "Y":dbl[]})  [unwired: 1 out]
    n119 = Unbundle(w322) -> (→"C2 Summed avg (mass)":cluster{dbl[], "Y":dbl[]})  [unwired: 1 out]
    n120 = property on="Channel 2  Summed Avg" class="WFGraph (strict)"("XScale.Offset"=w326) -> ()  [unwired: 2 in, 2 out]
    n121 = property on="Channel 1 Summed Avg" class="WFGraph (strict)"("XScale.Offset"=w329) -> ()  [unwired: 2 in, 2 out]
    n122 = Unbundle(w313) -> ("Cycle Count In"=→"Trace # (C1)":i32, "Cycle Count In"=→"Trace # (C2)":i32)
    n123 = event shown="[1] \"Save C1 Trace\": Value Change" {
      selector: _ -> [_ _ _ _ _ _]
      dyn-events: _ -> [_ _ _ _ _ _]
      timeout: 1 -> [_ _ _ _ _ _]
      tunnel: w347 -> [w354 w364 w374 w379 w382 w390]
      tunnel: [w354 w364 w374 w379 w382 w390] -> w346
      tunnel: w340 -> [w353 w363 w373 _ w388 w396]
      tunnel: [w353 w363 w373 T5 {"C1 Summed Waveform 2"={"t0"=timestamp(0 s since 1904-01-01), "dt"=1.0, "Y"=[]}, "C1 Summed Waveform 2"={"t0"=timestamp(0 s since 1904-01-01), "dt"=1.0, "Y"=[]}} ("Summed WFms In") w388 w396] -> w332
      tunnel: w315 -> [w352 w360 w370 w380 w387 w395]
      tunnel: [w352 w359 w369 w380 w387 w395] -> w320
      tunnel: w313 -> [w351 w362 w372 _ w386 w394]
      tunnel: [w351 w362 w372 w377 w385 w393] -> w341
      tunnel: w337 -> [w350 w361 w371 w376 w381 w389]
      tunnel: [w350 w361 w371 w376 w381 w389] -> w336
      tunnel: w319 -> [_ w358 w368 _ _ _]
      tunnel: "Default Data Directory" -> [_ w357 w367 _ _ _]
      tunnel: w318 -> [_ w355 w366 _ _ _]
      event Timeout {
        n124 = event-data() -> ()  [unwired: 1 in, 3 out]
      }
      event "Save C1 Trace": Value Change {
        w356 = u16 0 items=["C1", "C2"] ("Channel")
        n125 = event-data() -> ()  [unwired: 1 in, 6 out]
        n126 = call "save_summed_trace.vi"("start path"=w357, "Channel"=w356, "Complete Data cluster"=w355, "error in (no error)"=w360, "Variables Cluster"=w358) -> ("error out"=w359:errorcluster)  [unwired: 10 in]
      }
      event "Save C2 Trace": Value Change {
        w365 = u16 1 items=["C1", "C2"] ("Channel")
        n127 = event-data() -> ()  [unwired: 1 in, 6 out]
        n128 = call "save_summed_trace.vi"("start path"=w367, "Channel"=w365, "Complete Data cluster"=w366, "error in (no error)"=w370, "Variables Cluster"=w368) -> ("error out"=w369:errorcluster)  [unwired: 10 in]
      }
      event "Reset Summed Averages": Value Change {
        w378 = 0
        n129 = event-data() -> ()  [unwired: 1 in, 6 out]
        n130 = Bundle(w378, w378) -> (w377:cluster{i32, i32})  [unwired: 1 in]
      }
      event "C1 enabled": Value Change {
        n131 = event-data() -> ()  [unwired: 1 in, 6 out]
        n132 = Unbundle(w386) -> ("Cycle Count In"=w384:i32)  [unwired: 1 out]
        n133 = Bundle(0, "Cycle Count In"=w384) -> (w385:cluster{i32, "Cycle Count In":i32})  [unwired: 1 in]
      }
      event "C2 enabled": Value Change {
        n134 = event-data() -> ()  [unwired: 1 in, 6 out]
        n135 = Unbundle(w394) -> ("Cycle Count In"=w392:i32)  [unwired: 1 out]
        n136 = Bundle("Cycle Count In"=w392, 0) -> (w393:cluster{"Cycle Count In":i32, i32})  [unwired: 1 in]
      }
    }
  }
  n137 = while {
    tunnel: w64 -> [w418]
    tunnel: w57 -> [w422]
    shift-right: [w419] -> _
    shift-left: w53 -> [w411]
    tunnel: w39 -> [w416]
    tunnel: w38 -> [w415]
    tunnel: [w414] -> w46
    tunnel: [w413] -> w47
    tunnel: [w412] -> w42
    shift-right: [w398] -> _
    shift-left: w35 -> [w399]
    stop <- w417 stop-if-true
    n138 = call "measure_aquisition_time.vi"("Old Time / ms"=w399) -> ("New Time / ms"=w398:u32, "Aqusition Time / ms"=→"Raw Data Processing  Exectuion Time / ms":u32)  [unwired: 12 in, 1 out]
    n139 = call "raw_Q_to_avg_Q.vi"("scope Q data"=w418, "avg_Q_data"=w422, "Variables Cluster"=w411) -> ("avg_Q_data out"=w420:T9, "Complete Data Out"=w410:T13, "error out"=w417:errorcluster)  [unwired: 10 in]
    n140 = Lossy Enqueue Element(queue=w416, element=w411, error in (no error)=w415) -> (queue out=w414:refnum<queue>, error out=w413:errorcluster)  [unwired: 2 out]
    n141 = call "prep_plotting_data.vi"("Plotting Data"=w410) -> ("C1 (time)"=w409:T14, "C2 (time)"=w406:T14, "C1 (mass)"=w402:cluster{dbl, cluster{dbl[], "Y":dbl[]}}, "C2 (mass)"=w401:cluster{dbl, cluster{dbl[], "Y":dbl[]}})  [unwired: 4 in]
    n142 = Unbundle(w401) -> (→"C2 Raw (mass)":cluster{dbl[], "Y":dbl[]})  [unwired: 1 out]
    n143 = Unbundle(w406) -> ("offset"=w405:dbl, "C1 Summed Waveform 2"=→"Channel 1 Raw":waveform(dbl))
    n144 = Unbundle(w409) -> ("offset"=w408:dbl, "C1 Summed Waveform 2"=→"Channel 2 Raw":waveform(dbl))
    n145 = Unbundle(w402) -> (→"C1 Raw (mass)":cluster{dbl[], "Y":dbl[]})  [unwired: 1 out]
    n146 = property on="Channel 2 Raw" class="WFGraph (strict)"("XScale.Offset"=w408) -> ()  [unwired: 2 in, 2 out]
    n147 = property on="Channel 1 Raw" class="WFGraph (strict)"("XScale.Offset"=w405) -> ()  [unwired: 2 in, 2 out]
    n148 = event shown="[0] Timeout" {
      selector: _ -> [_ _ _ _ _ _]
      dyn-events: _ -> [_ _ _ _ _ _]
      timeout: 1 -> [_ _ _ _ _ _]
      tunnel: w420 -> [w423 w427 w433 w437 w441 w445]
      tunnel: w411 -> [w424 w430 w436 w440 w444 w448]
      tunnel: [w424 w429 w435 w439 w443 w447] -> w419
      tunnel: [w423 w426 w432 w437 w441 w445] -> w412
      event Timeout {
        n149 = event-data() -> ()  [unwired: 1 in, 3 out]
      }
      event "RT Avg Trace #": Value Change {
        n150 = event-data() -> ("NewVal"=w428:i32)  [unwired: 1 in, 2 out]
        n151 = Bundle By Name(cluster=w430, "RT Avg Trace #"=w428) -> (w429:T6)
        n152 = call "flush_avg_queues.vi"("Combo Box"="RT Avg", "avg_Q_data in"=w427) -> ("avg_Q_data out"=w426:T9)  [unwired: 13 in]
      }
      event "Summed Trace #": Value Change {
        n153 = event-data() -> ("NewVal"=w434:i32)  [unwired: 1 in, 2 out]
        n154 = Bundle By Name(cluster=w436, "Summed Avg Trace #"=w434) -> (w435:T6)
        n155 = call "flush_avg_queues.vi"("Combo Box"="Summed Avg", "avg_Q_data in"=w433) -> ("avg_Q_data out"=w432:T9)  [unwired: 13 in]
      }
      event "Gradient": Value Change {
        n156 = event-data() -> ("NewVal"=w438:dbl)  [unwired: 1 in, 5 out]
        n157 = Bundle By Name(cluster=w440, "Gradient"=w438) -> (w439:T6)
      }
      event "Intercept": Value Change {
        n158 = event-data() -> ("NewVal"=w442:dbl)  [unwired: 1 in, 5 out]
        n159 = Bundle By Name(cluster=w444, "Intercept"=w442) -> (w443:T6)
      }
      event "Mass Conversion": Value Change {
        n160 = event-data() -> ("NewVal"=w446:bool)  [unwired: 1 in, 5 out]
        n161 = Bundle By Name(cluster=w448, "Mass Conversion"=w446) -> (w447:T6)
      }
    }
  }
  n162 = while {
    tunnel: w57 -> [w471]
    tunnel: [w472] -> _
    tunnel: w39 -> [w470]
    tunnel: w38 -> [w469]
    shift-right: [w466] -> _
    shift-left: w45 -> [w467]
    stop <- w451 stop-if-true
    n163 = Preview Queue Element(queue=w470, error in (no error)=w469) -> (element=w464:T6, error out=w449:errorcluster)  [unwired: 1 in, 2 out]
    n164 = call "extract_avg_data.vi"("Combo Box"="RT Avg", "avg_Q_data in"=w471) -> ("avg_Q_data out"=w472:T9, "RT Avg Data Out"=w465:T15, "error out"=w452:errorcluster)  [unwired: 10 in, 1 out]
    n165 = call "generate_RT_average.vi"("Data In"=w465, "Variables Cluster"=w464) -> ("Complete Data Out"=w463:T13, "error out"=w450:errorcluster)  [unwired: 12 in]
    n166 = call "prep_plotting_data.vi"("Plotting Data"=w463) -> ("C1 (time)"=w462:T14, "C2 (time)"=w459:T14, "C1 (mass)"=w456:cluster{dbl, cluster{dbl[], "Y":dbl[]}}, "C2 (mass)"=w455:cluster{dbl, cluster{dbl[], "Y":dbl[]}})  [unwired: 4 in]
    n167 = Compound Arithmetic op=OR(w452, w449, w450) -> (w451:bool)
    n168 = call "measure_aquisition_time.vi"("Old Time / ms"=w467) -> ("New Time / ms"=w466:u32, "Aqusition Time / ms"=→"RT Average Exectuion Time / ms":u32)  [unwired: 12 in, 1 out]
    n169 = Unbundle(w455) -> (→"C2 RT avg (mass)":cluster{dbl[], "Y":dbl[]})  [unwired: 1 out]
    n170 = Unbundle(w456) -> (→"C1 RT avg (mass)":cluster{dbl[], "Y":dbl[]})  [unwired: 1 out]
    n171 = Unbundle(w459) -> ("offset"=w458:dbl, "C1 Summed Waveform 2"=→"Channel 2 RT Avg":waveform(dbl))
    n172 = Unbundle(w462) -> ("offset"=w461:dbl, "C1 Summed Waveform 2"=→"Channel 1 RT Avg":waveform(dbl))
    n173 = property on="Channel 1 RT Avg" class="WFGraph (strict)"("XScale.Offset"=w461) -> ()  [unwired: 2 in, 2 out]
    n174 = property on="Channel 2 RT Avg" class="WFGraph (strict)"("XScale.Offset"=w458) -> ()  [unwired: 2 in, 2 out]
  }
  n175 = call "delete_scope_data_Qs.vi"("scope Q data"=w61) -> ()  [unwired: 14 in, 1 out]
  n176 = call <instrlib>:"niScope Close.vi"("instrument handle"=w66, "error in"=w65) -> ("error out"=w34:errorcluster)  [unwired: 13 in]
  n177 = call "del_avg_Qs.vi"("avg_Q_data"=w42) -> ()  [unwired: 14 in, 1 out]
  n178 = Current VI's Path() -> (path=w32:path)
  n179 = Release Queue(queue=w46, error in (no error)=w47) -> ()  [unwired: 1 in, 3 out]
  n180 = call "save_scope_config.vi"("Current VI's Path"=w32, "Save File Type"=w31, "Controls cluster"=w33, "error in"=w34) -> ()  [unwired: 10 in, 2 out]
